vi "get_wavelength.vi"(8 "error in (no error)":errorcluster, 11 "LightSourceAN191011Chameleon in":refnum<class "LightSourceAN191011Chameleon.lvclass">) -> (0 "error out":errorcluster, 2 "wavelength":dbl[unit], 3 "LightSourceAN191011Chameleon out":refnum<class "LightSourceAN191011Chameleon.lvclass">)   [LabVIEW 2011, in "LightSourceAN191011Chameleon.lvclass"]
uses:
  LightSourceAN191011Chameleon.lvclass
  LightSourceAN191011Chameleon.lvclass/LightSourceAN191011Chameleon.ctl
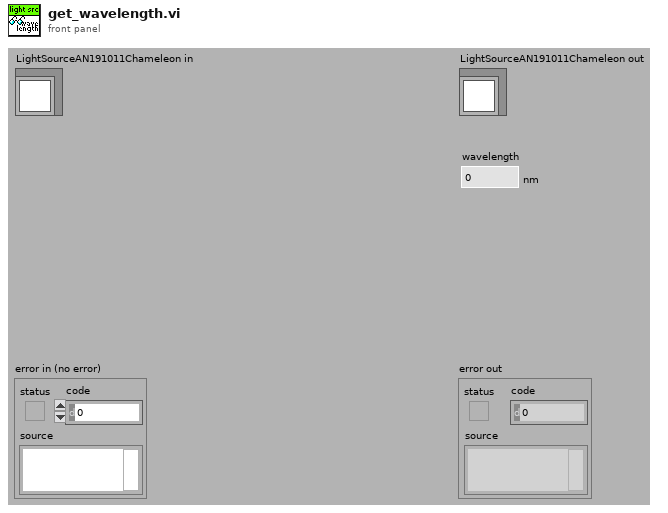
[diagram p1: front panel]
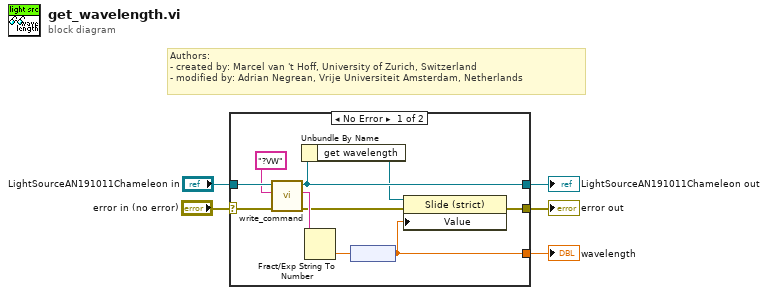
[diagram p0: block diagram]
diagram:
  # "Authors: \n- created by: Marcel van 't Hoff, University of Zurich, Switzerland\n- modified by: Adrian Negrean, Vrije Universiteit Amsterdam, Netherlands"
  n1 = case shown="No Error" "error in (no error)" {
    selector: "error in (no error)" -> [w14 w17]
    tunnel: [w6 w17] -> w4
    tunnel: [w10 w16] -> w2
    tunnel: "LightSourceAN191011Chameleon in" -> [w15 w16]
    tunnel: [w9 _] -> w1
    frame No Error {
      n2 = call-dynamic "write_command.vi"("error in (no error)"=w14, "string to write"="?VW", "LightSourceAN191011Chameleon in"=w15) -> ("error out"=w7:errorcluster, "read string"=w12:string, "LightSourceAN191011Chameleon out"=w10:refnum<class "LightSourceAN191011Chameleon.lvclass">)  [unwired: 6 in]
      n3 = Unbundle By Name(w10) -> ("get wavelength"=w8:refnum<vi>)
      n4 = Fract/Exp String To Number(string=w12) -> (number=w11:dbl)  [unwired: 3 in, 1 out]
      n5 = node(w11) -> (w9:dbl[unit])
      n6 = property class="Slide (strict)"(reference=w8, error in=w7, "Value"=w9) -> (error out=w6:errorcluster)  [unwired: 1 out]
    }
    frame Error {
    }
  }
  "error out" <- w4
  "LightSourceAN191011Chameleon out" <- w2
  "wavelength" <- w1
